vi "GCMLogGlobals.vi"() -> ()   [LabVIEW 2014, in "GCMLog.lvclass"]
uses:
  GCMLog.lvclass
panel:
  in  "LogPath":path
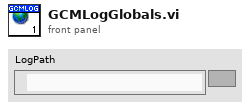
[diagram p1: front panel]
diagram:
